vi "Optics_Close_COM.VI"(8 "Error in":errorcluster, 11 "VISA":refnum<visa-resource-name>) -> (0 "Error out":errorcluster)   [LabVIEW 2021]
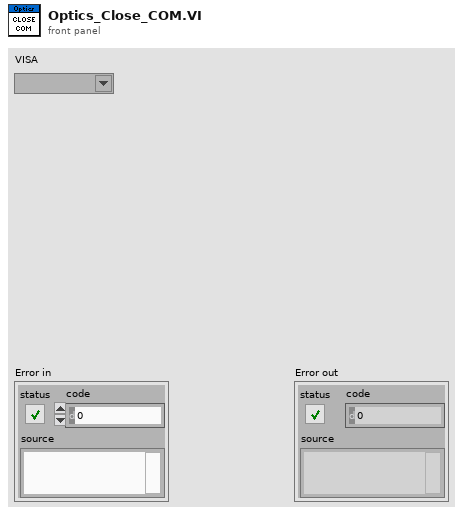
[diagram p1: front panel]
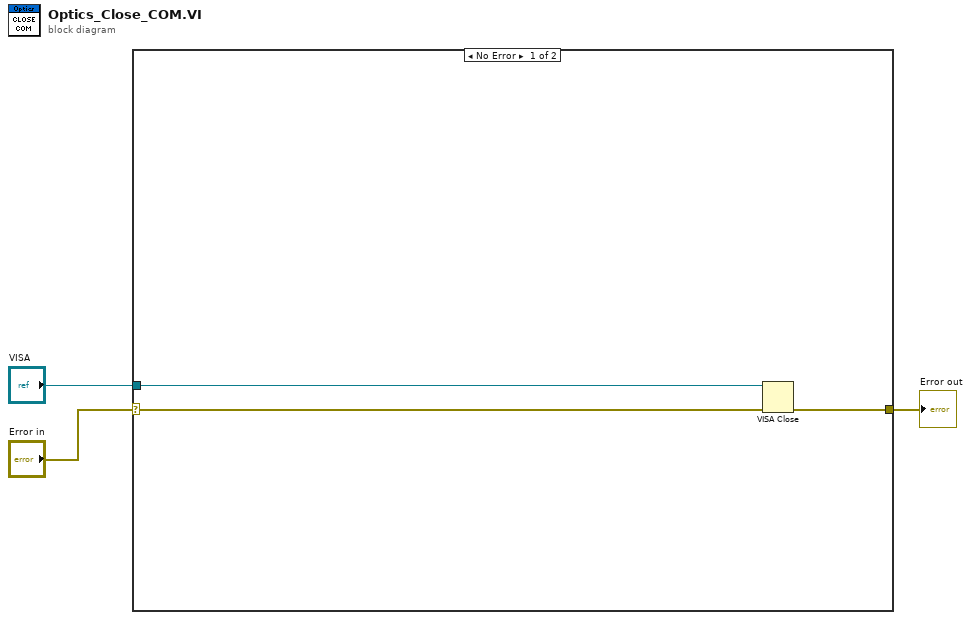
[diagram p0: block diagram]
diagram:
  n1 = case shown="No Error" "Error in" {
    selector: "Error in" -> [w5 w7]
    tunnel: [w6 w7] -> w3
    tunnel: "VISA" -> [w4 _]
    frame No Error {
      n2 = VISA Close(VISA resource name=w4, error in (no error)=w5) -> (error out=w6:errorcluster)
    }
    frame Default {
    }
  }
  "Error out" <- w3
